vi "FeedbackDecode_PtPtMeanStd.vi"(1 "Initialize":bool, 2 "Array":dbl[](array[numeric])=[0.0]) -> (5 "Mean":dbl[](array[numeric]), 6 "Std":dbl[](array[numeric]))   [LabVIEW 2020]
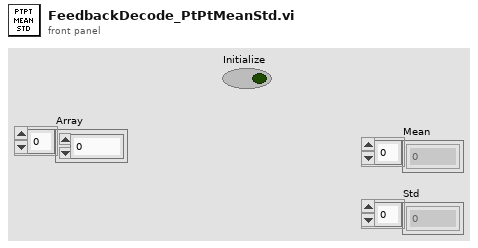
[diagram p1: front panel]
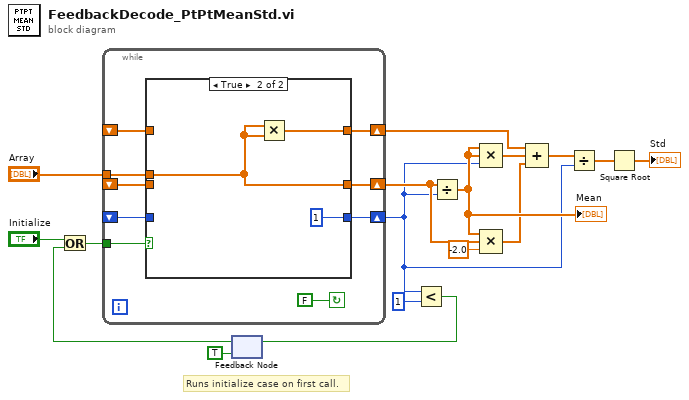
[diagram p0: block diagram]
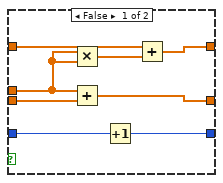
[diagram p2: hidden frame]
diagram:
  # "Runs initialize case on first call."
  n1 = feedback #1(TRUE) -> (w6:bool)
  n2 = Or(x="Initialize", y=w6) -> (x .or. y?=w8:bool)
  n3 = while {
    shift-right: [w25] -> w4
    shift-left: _ -> [w24]
    shift-right: [w19] -> w15
    shift-left: _ -> [w23]
    shift-right: [w20] -> w16
    shift-left: _ -> [w21]
    tunnel: "Array" -> [w22]
    tunnel: w8 -> [w18]
    stop <- FALSE continue-if-true
    n4 = case shown="True" w18 {
      tunnel: [w34 1 ("y")] -> w25
      tunnel: w24 -> [w33 _]
      tunnel: w23 -> [w32 _]
      tunnel: w22 -> [w31 w36]
      tunnel: w21 -> [w30 _]
      tunnel: [w29 w37] -> w20
      tunnel: [w28 w36] -> w19
      frame False {
        n5 = Multiply(x=w31, y=w31) -> (x*y=w27:dbl[])
        n6 = Add(x=w31, y=w32) -> (x+y=w28:dbl[])
        n7 = Increment(x=w33) -> (x+1=w34:i32)
        n8 = Add(x=w30, y=w27) -> (x+y=w29:dbl[])
      }
      frame True {
        n9 = Multiply(x=w36, y=w36) -> (x*y=w37:dbl[])
      }
    }
  }
  n10 = Less?(x=w4, y=1) -> (x < y?=w7:bool)
  n11 = feedback-in #1(w7) -> ()
  n12 = Divide(x=w15, y=w4) -> (x/y=w14:dbl[])
  "Mean" <- w14
  n13 = Compound Arithmetic op=MULTIPLY(w14, w14, w4) -> (w17:dbl[])
  n14 = Compound Arithmetic op=MULTIPLY(w14, w15, -2.0) -> (w12:dbl[])
  n15 = Compound Arithmetic op=ADD(w16, w17, w12) -> (w11:dbl[])
  n16 = Divide(x=w11, y=w4) -> (x/y=w2:dbl[])
  n17 = Square Root(x=w2) -> (sqrt(x)=→"Std":dbl[])
